vi "ArdnoValveArray2Control.vi"(10 "Cluster in":refnum<vi>, 11 "ValveStates":bool[](array[boolean])) -> ()   [LabVIEW 2018]
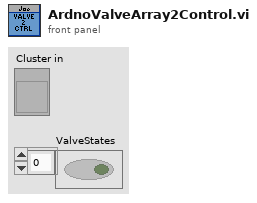
[diagram p1: front panel]
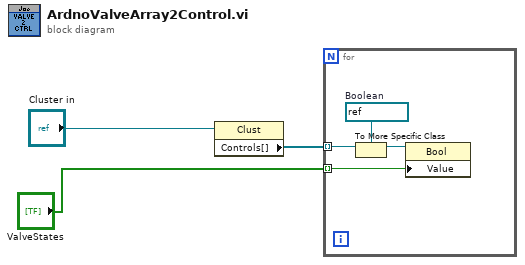
[diagram p0: block diagram]
diagram:
  n1 = property class="Clust"(reference="Cluster in") -> ("Controls[]"=w2:refnum<vi>[])  [unwired: 1 in, 2 out]
  n2 = for {
    tunnel: w2 -> [w7] mode=indexing
    tunnel: "ValveStates" -> [w4] mode=indexing
    w5 = refnum<vi> refnum  # Boolean
    n3 = To More Specific Class(target class=w5, reference=w7) -> (specific class reference=w6:refnum<vi>)  [unwired: 1 in, 1 out]
    n4 = property class="Bool"(reference=w6, "Value"=w4) -> ()  [unwired: 1 in, 2 out]
  }
